vi "Exit.vi"(8 "error in (no error)":errorcluster, 11 "Old State":refnum<class "Cursor.lvclass">) -> (0 "error out":errorcluster, 3 "New State":refnum<class "Cursor.lvclass">)   [LabVIEW 2020, in "Keypad.lvlib" / "Cursor.lvclass"]
doc: "This is an abstract method. Override this method to define the behavior when you leave the state."
uses:
  Cursor.lvclass
  Keypad/Keypad.lvclass
  Type Def - Cursor Display.ctl
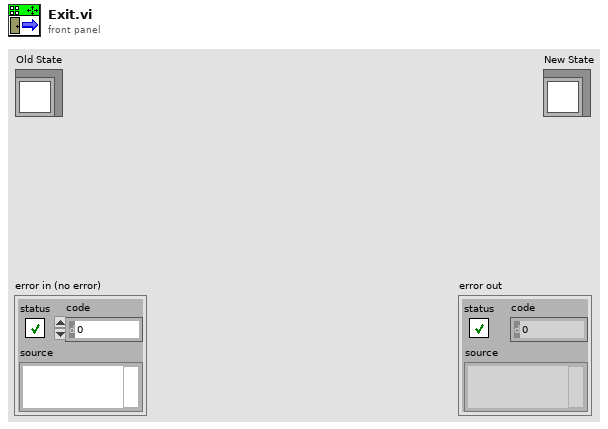
[diagram p1: front panel]
types:
  T1 = typedef "Type Def - Cursor Display.ctl" = cluster{"Up":bool, "Left":bool, "Ctr":bool, "Right":bool, "Down":bool}
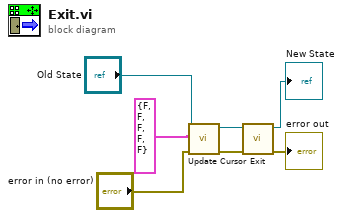
[diagram p0: block diagram]
diagram:
  n1 = call "Update Cursor.vi"("error in (no error)"="error in (no error)", "Cursor"=T1 {"Up"=FALSE, "Left"=FALSE, "Ctr"=FALSE, "Right"=FALSE, "Down"=FALSE}, "Keypad in"="Old State") -> ("error out"=w3:errorcluster, "Keypad out"=w4:refnum<class "Cursor.lvclass">)  [unwired: 7 in]
  n2 = call-parent "Exit.vi"("error in (no error)"=w3, "Old State"=w4) -> ("error out"=→"error out":errorcluster, "New State"=→"New State":refnum<class "Cursor.lvclass">)  [unwired: 8 in]
